vi "Sigmoid_kernel.vi"(8 "error in":errorcluster caption="entrée d'erreur", 9 "Y":string[][](array[string]), 10 "X":string[][](array[string]), 11 "sigmoid_kernel":cluster{"gamma":string, "coef0":dbl}={"gamma"="None", "coef0"=1.0}) -> (0 "error out":errorcluster caption="sortie d'erreur", 3 "Data":T1)   [LabVIEW 2020]
doc: "Compute the sigmoid kernel between X and Y :\n\nK(X, Y) = tanh(gamma <X, Y> + coef0)\n\nParameters : \n\n- X : ndarray of shape (n_samples_1, n_features)\n\n- Y : ndarray of shape (n_samples_2, n_features)\n\n- gamma : float, default None\nIf None, defaults to 1.0 / n_features\n\n- coef0 : float, default 1\n\nReturns : \n\n- Gram matrix : array of shape (n_samples_1, n_samples_2)"
uses:
  Sigmoid_kernel.lvclass
panel:
  out "Sigmoid_kernel.lvclass":refnum<class "Sigmoid_kernel.lvclass">
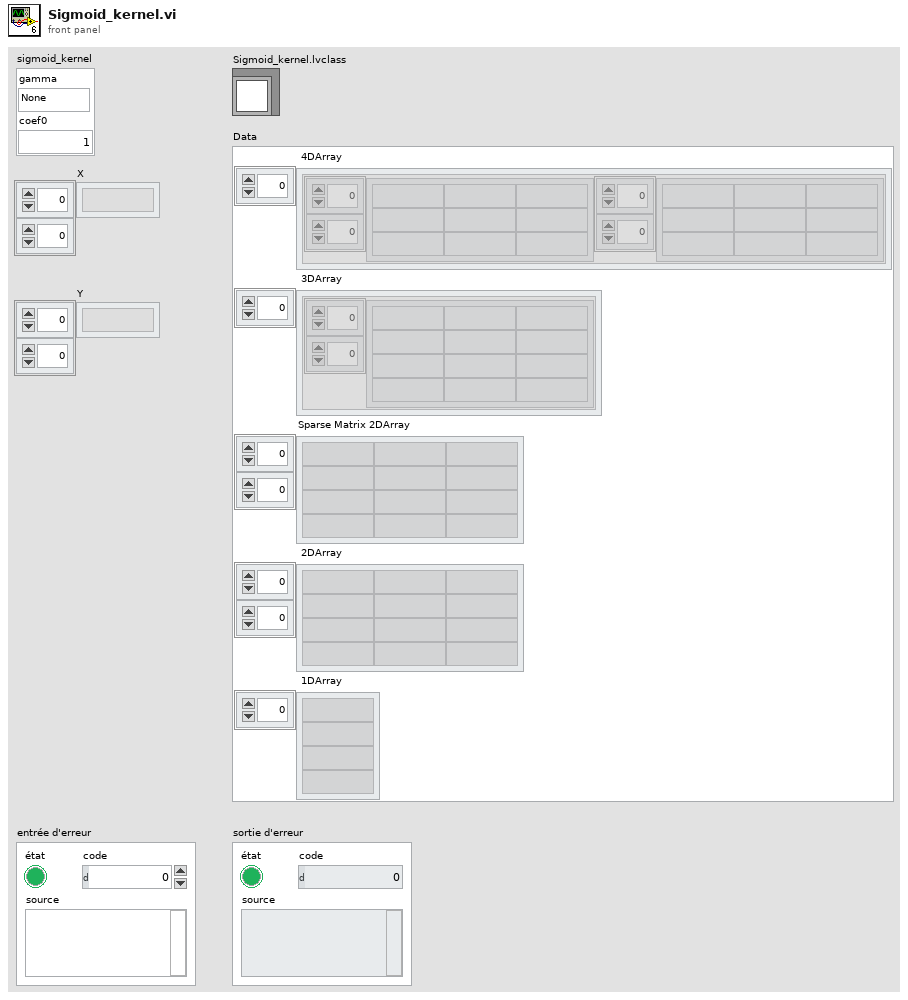
[diagram p1: front panel]
types:
  T1 = cluster{" 4DArray":cluster{"1":string[][], "2":string[][]}[], " 3DArray":cluster{"Tableau":string[][]}[], "Sparse Matrix 2DArray":string[][], " 2DArray":string[][], " 1DArray":string[]}
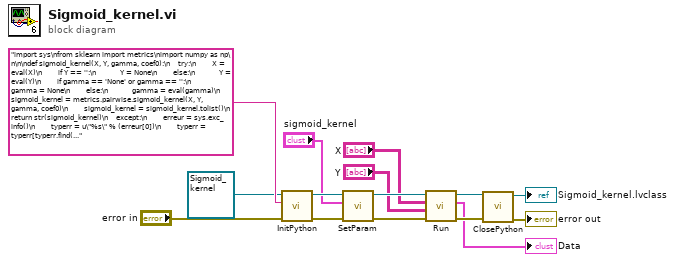
[diagram p0: block diagram]
diagram:
  n1 = call-dynamic "InitPython.vi"("error in (no error)"="error in", "Python Instruction"="import sys\nfrom sklearn import metrics\nimport numpy as np\n\n\ndef sigmoid_kernel(X, Y, gamma, coef0):\n    try:\n        X = eval(X)\n        if Y == '':\n            Y = None\n        else:\n            Y = eval(Y)\n        if gamma == 'None' or gamma == '':\n            gamma = None\n        else:\n            gamma = eval(gamma)\n        sigmoid_kernel = metrics.pairwise.sigmoid_kernel(X, Y, gamma, coef0)\n        sigmoid_kernel = sigmoid_kernel.tolist()\n        return str(sigmoid_kernel)\n    except:\n        erreur = sys.exc_info()\n        typerr = u\"%s\" % (erreur[0])\n        typerr = typerr[typerr.find(\"'\")+1:typerr.rfind(\"'\")]\n        msgerr = u\"%s\" % (erreur[1])\n        message = str('/!\\\\ {0} : {1}'. format(typerr,msgerr))\n        return message", "Scikit-learn en entrée"=refnum<class "Sigmoid_kernel.lvclass"> refnum ("Sigmoid_kernel.lvclass")) -> ("error out"=w12:errorcluster, "Scikit-learn en sortie"=w11:refnum<class "Sigmoid_kernel.lvclass">)  [unwired: 7 in]
  n2 = call-dynamic "SetParam.vi"("error in (no error)"=w12, "sigmoid_kernel"="sigmoid_kernel", "Sigmoid_kernel.lvclass"=w11) -> ("error out"=w6:errorcluster, "Sigmoid_kernel.lvclass"=w7:refnum<class "Sigmoid_kernel.lvclass">)  [unwired: 7 in]
  n3 = call-dynamic "Run.vi"("error in (no error)"=w6, "Y"="Y", "X"="X", "Sigmoid_kernel.lvclass"=w7) -> ("error out"=w9:errorcluster, "Data"=→"Data":T1, "Sigmoid_kernel.lvclass"=w10:refnum<class "Sigmoid_kernel.lvclass">)  [unwired: 5 in]
  n4 = call-dynamic "ClosePython.vi"("error in (no error)"=w9, "Scikit-learn en entrée"=w10) -> ("error out"=→"error out":errorcluster, "Scikit-learn en sortie"=→"Sigmoid_kernel.lvclass":refnum<class "Sigmoid_kernel.lvclass">)  [unwired: 8 in]
